vi "Greatest Common Prime Factor (GCPF)-scalar input.vi"(8 "error in (no error)":errorcluster, 10 "y":i32, 11 "x":i32) -> (0 "error out":errorcluster, 2 "T = x and y are relatively prime":bool, 3 "Greatest Common Prime Factor (GCPF)":i32)   [LabVIEW 2021, in "Numeric Utilities.lvlib"]
uses:
  Numeric Utilities.lvlib
panel:
  out "Loop iteration":i32
  out "Common prime divisors of x and y":i32[](array[numeric])
  out "T = common prime divisor":bool
  out "Prime factors of y":i32[](array[numeric])
  out "Prime factors of x":i32[](array[numeric])
  # "Development\ncontrols/indicators useful for development and testing, but which are not outputs of the VI"
  # "Input\nInputs to the VI"
  # "Output\nOutputs of the VI"
  # "Description\n\nBlank VI with error handling case. \n\nSummarize the use of this VI in this space."
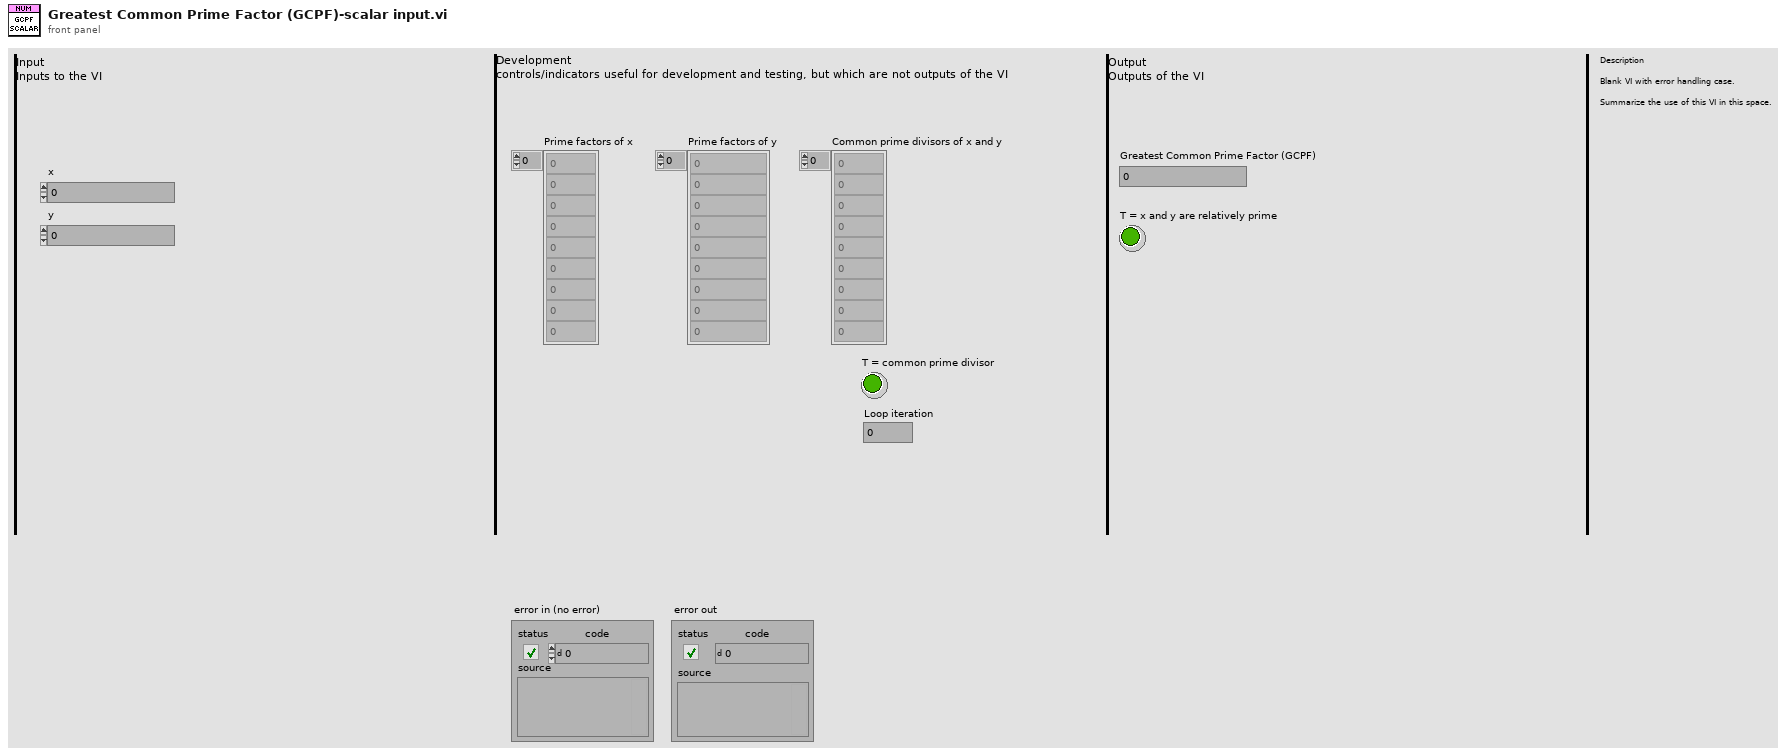
[diagram p1: front panel]
types:
  T1 = typedef "Numeric Utilities.lvlib/Factors cluster.ctl" = cluster{"Factor":i32, "Power":i32}
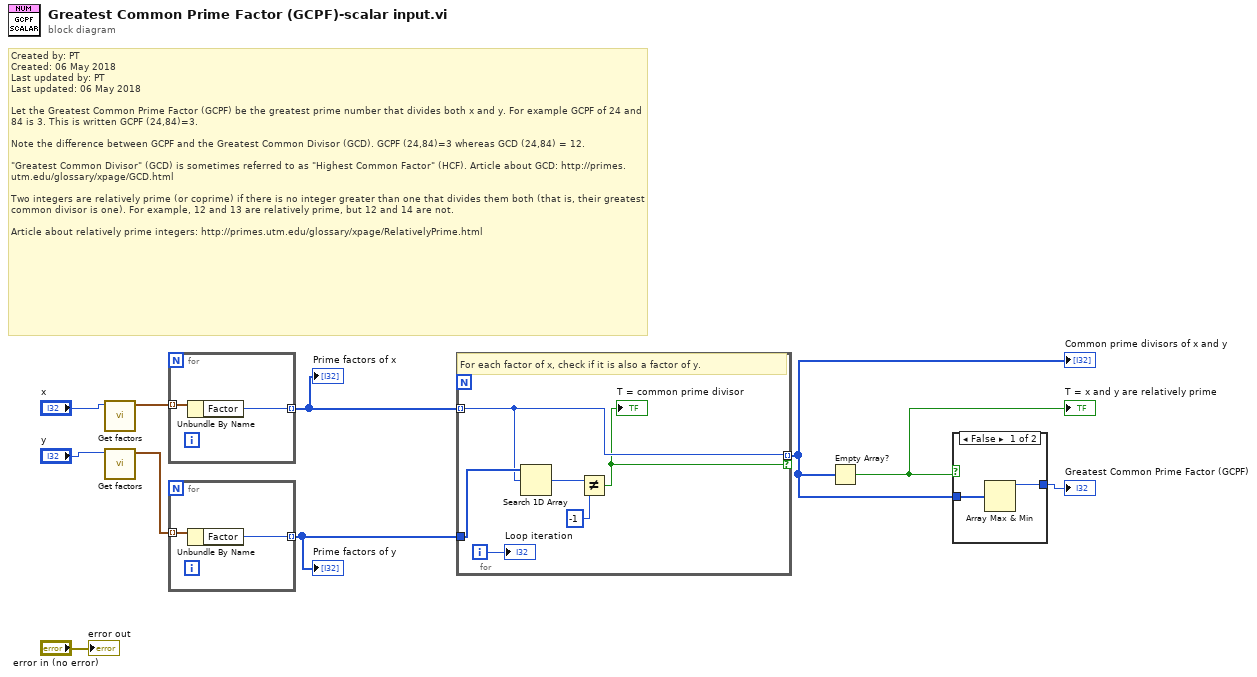
[diagram p0: block diagram]
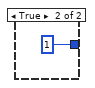
[diagram p2: hidden frame]
diagram:
  # "Created by: PT\nCreated: 06 May 2018\nLast updated by: PT\nLast updated: 06 May 2018\n\nLet the Greatest Common Prime Factor (GCPF) be the greatest prime number that divides both x and y. For example GCPF of 24 and 84 is 3. This is written GCPF (24,84)=3.\n\nNote the difference between GCPF and the Greatest Common Divisor (GCD). GCPF (24,84)=3 whereas GCD (24,84) = 12.\n\n\"Greatest Common Divisor\" (GCD) is sometimes referred to as \"Highest Common Factor\" (HCF). Article about GCD: http://primes.utm.edu/glossary/xpage/GCD.html\n\nTwo integers are relatively prime (or coprime) if there is no integer greater than one that divides them both (that is, their greatest common divisor is one). For example, 12 and 13 are relatively prime, but 12 and 14 are not.\n\nArticle about relatively prime integers: http://primes.utm.edu/glossary/xpage/RelativelyPrime.html"
  n1 = call "Get factors.vi"("x"="x") -> ("Factors out"=w7:T1[])  [unwired: 5 in, 5 out]
  n2 = call "Get factors.vi"("x"="y") -> ("Factors out"=w6:T1[])  [unwired: 5 in, 5 out]
  n3 = for {
    tunnel: w7 -> [w12] mode=indexing
    tunnel: [w11] -> w5 mode=indexing
    n4 = Unbundle By Name(w12) -> ("Factor"=w11:i32)
  }
  "Prime factors of x" <- w5
  n5 = for {
    tunnel: w6 -> [w14] mode=indexing
    tunnel: [w13] -> w4 mode=indexing
    n6 = Unbundle By Name(w14) -> ("Factor"=w13:i32)
  }
  "Prime factors of y" <- w4
  n7 = for {
    tunnel: w5 -> [w17] mode=indexing
    tunnel: w4 -> [w20]
    tunnel: [w17] -> w2 mode=indexing if=w16
    i -> [w15]
    # "For each factor of x, check if it is also a factor of y."
    n8 = Search 1D Array(1D array=w20, element=w17) -> (index of element=w19:i32)  [unwired: 1 in]
    n9 = Not Equal?(x=w19, y=-1) -> (x != y?=w16:bool)
    "T = common prime divisor" <- w16
    "Loop iteration" <- w15
  }
  "Common prime divisors of x and y" <- w2
  n10 = Empty Array?(array=w2) -> (empty?=w1:bool)
  "T = x and y are relatively prime" <- w1
  n11 = case shown="False" w1 {
    tunnel: w2 -> [w22 _]
    tunnel: [w21 1] -> w3
    frame False {
      n12 = Array Max & Min(array=w22) -> (max value=w21:i32)  [unwired: 3 out]
    }
    frame True {
    }
  }
  "Greatest Common Prime Factor (GCPF)" <- w3
  "error out" <- "error in (no error)"
